vi "基于Lab颜色空间的自适应分割算法.vi"(11 "火焰占比系数":dbl(slide)=0.9 min=0.0 max=1.0 step=0.05 scale=0.0..1.0 scale format="%1.2f") -> ()   [LabVIEW 2018]
doc: "This example shows how to open, read, and display an AVI file in NI Vision. The VI reads the frames per second property and plays the images back at the rate specified by the AVI file."
uses:
  <vilib>/vision/NI_Vision_Development_Module.lvlib
  Dll/fire_Otsu.dll
panel:
  out "导入像素当量":bool
  in  "?":bool
  out "叠加实际字符串":string
  out "单帧实际字符串":string
  out "叠加像素字符串":string
  out "单帧像素字符串":string
  out "循环截止":bool
  in  "取消按钮":bool
  out "火焰帧数":string
  in  "单帧回看":bool
  out "叠加部分":string
  out "单帧部分":string
  in  "返回":bool
  out "火焰分割":T1(plugin-control)
  out "单幅画面":T1(plugin-control) caption="单帧画面"
  out "Progress Bar":i32(slide) max=241 scale=-1.1..241.0
  in  "程序停止":bool
  out "原图":T1(plugin-control)
  out "火焰叠加":T1(plugin-control)
  # "Lab颜色空间的最大类间方法火焰分割"
  # "火焰参数"
  # "参\n数\n设\n置"
  # "说明：\n火焰实际面积的单位为标定时的设定的单位，若未进行标注，则不显示实际尺寸。"
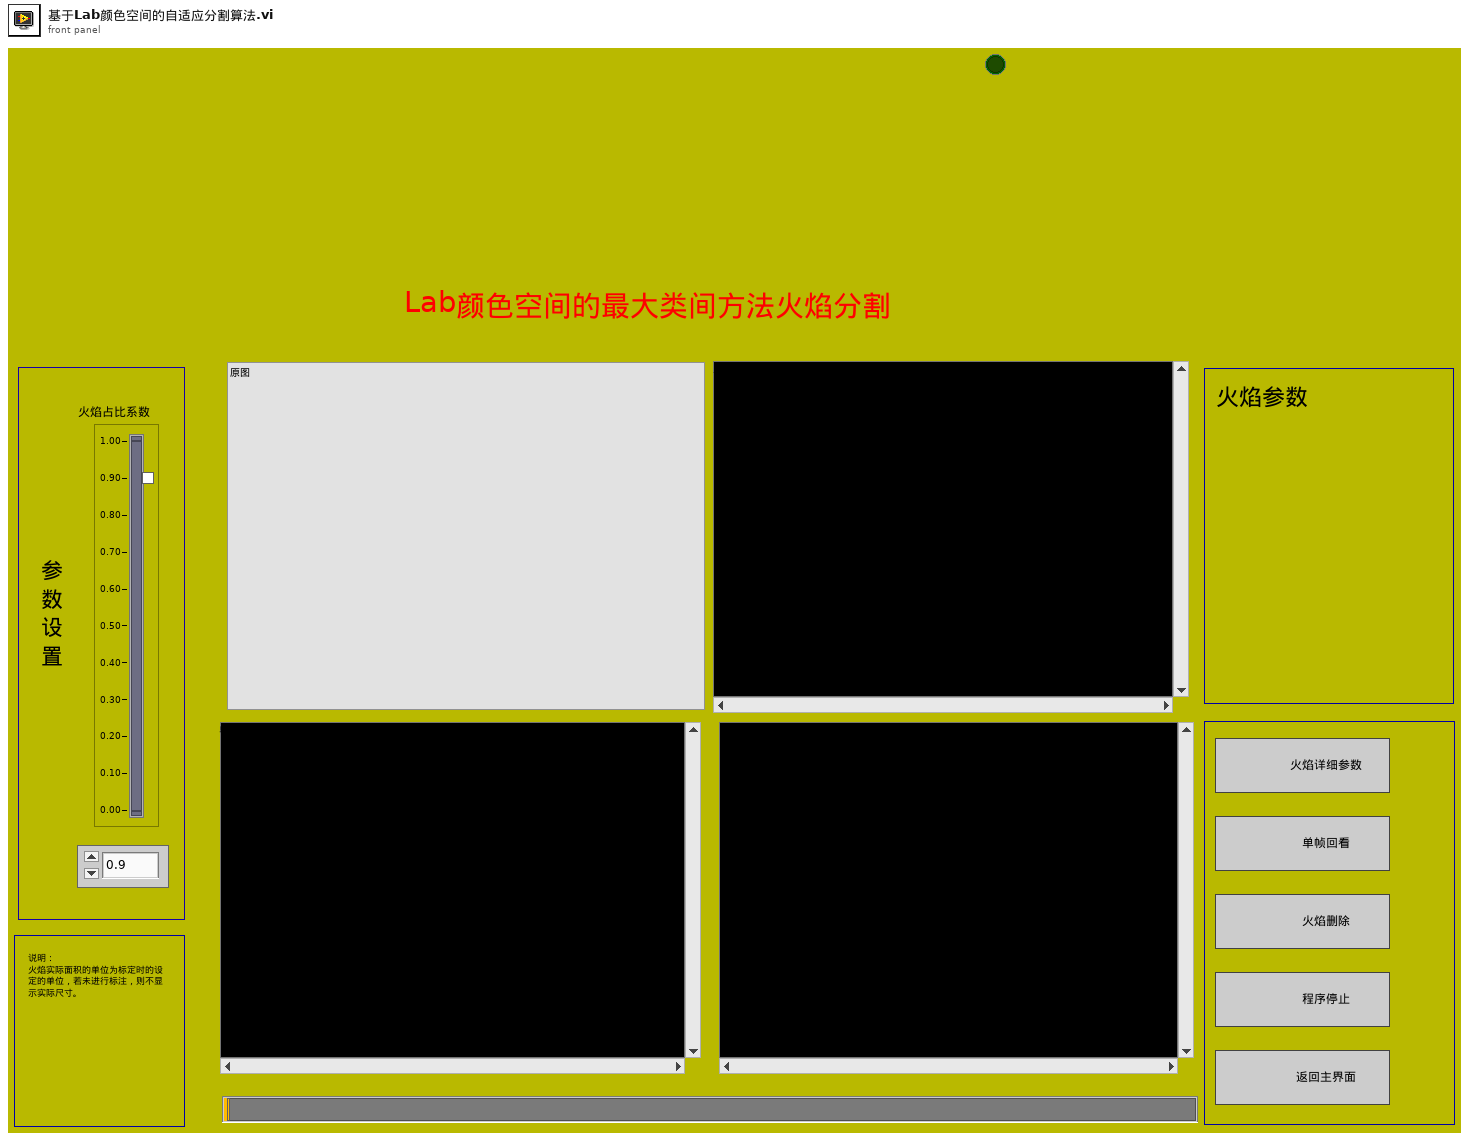
[diagram p1: front panel]
types:
  T1 = typedef "IMAQ Image.ctl" = refnum<image>
  T2 = enum8{"Enabled", "Disabled", "Disabled and Grayed Out"}
  T3 = cluster{"X Size":i32, "Y Size":i32, "% Tolerance":i32}
  T4 = enum32{"Invalid", "Standard", "Closed", "Hidden", "Minimized", "Maximized"}
  T5 = typedef "Image Type" = u32
  T6 = cluster{"Width":u32, "Height":u32, "Frames Per Second":u32, "Codec":string, "Has Data":bool}
  T7 = typedef "IMAQ AVI2 Refnum.ctl" = refnum<k20>
  T8 = typedef "ROI Descriptor" = cluster{"Global Rectangle":i32[], "Contours":cluster{"ID":enum32{"External", "Internal"}, "Type":u32, "Coordinates":i32[]}[]}
  T9 = cluster{"Area":dbl, "Number of Holes":dbl, "Bounding Rect":cluster{"Left":dbl, "Top":dbl, "Right":dbl, "Bottom":dbl}, "Center of Mass":cluster{"X":dbl, "Y":dbl}, "Orientation":dbl, "Dimensions":cluster{"Width":dbl, "Height":dbl}}[]
  T10 = cluster{"Particle Reports (Pixels)[0]":cluster{"Area":dbl, "Number of Holes":dbl, "Bounding Rect":cluster{"Left":dbl, "Top":dbl, "Right":dbl, "Bottom":dbl}, "Center of Mass":cluster{"X":dbl, "Y":dbl}, "Orientation":dbl, "Dimensions":cluster{"Width":dbl, "Height":dbl}}, "Particle Reports (Pixels)[1]":cluster{"Area":dbl, "Number of Holes":dbl, "Bounding Rect":cluster{"Left":dbl, "Top":dbl, "Right":dbl, "Bottom":dbl}, "Center of Mass":cluster{"X":dbl, "Y":dbl}, "Orientation":dbl, "Dimensions":cluster{"Width":dbl, "Height":dbl}}, "Particle Reports (Pixels)[2]":cluster{"Area":dbl, "Number of Holes":dbl, "Bounding Rect":cluster{"Left":dbl, "Top":dbl, "Right":dbl, "Bottom":dbl}, "Center of Mass":cluster{"X":dbl, "Y":dbl}, "Orientation":dbl, "Dimensions":cluster{"Width":dbl, "Height":dbl}}, "Particle Reports (Pixels)[3]":cluster{"Area":dbl, "Number of Holes":dbl, "Bounding Rect":cluster{"Left":dbl, "Top":dbl, "Right":dbl, "Bottom":dbl}, "Center of Mass":cluster{"X":dbl, "Y":dbl}, "Orientation":dbl, "Dimensions":cluster{"Width":dbl, "Height":dbl}}, "Particle Reports (Pixels)[4]":cluster{"Area":dbl, "Number of Holes":dbl, "Bounding Rect":cluster{"Left":dbl, "Top":dbl, "Right":dbl, "Bottom":dbl}, "Center of Mass":cluster{"X":dbl, "Y":dbl}, "Orientation":dbl, "Dimensions":cluster{"Width":dbl, "Height":dbl}}, "Particle Reports (Pixels)[5]":cluster{"Area":dbl, "Number of Holes":dbl, "Bounding Rect":cluster{"Left":dbl, "Top":dbl, "Right":dbl, "Bottom":dbl}, "Center of Mass":cluster{"X":dbl, "Y":dbl}, "Orientation":dbl, "Dimensions":cluster{"Width":dbl, "Height":dbl}}, "Particle Reports (Pixels)[6]":cluster{"Area":dbl, "Number of Holes":dbl, "Bounding Rect":cluster{"Left":dbl, "Top":dbl, "Right":dbl, "Bottom":dbl}, "Center of Mass":cluster{"X":dbl, "Y":dbl}, "Orientation":dbl, "Dimensions":cluster{"Width":dbl, "Height":dbl}}, "Particle Reports (Pixels)[7]":cluster{"Area":dbl, "Number of Holes":dbl, "Bounding Rect":cluster{"Left":dbl, "Top":dbl, "Right":dbl, "Bottom":dbl}, "Center of Mass":cluster{"X":dbl, "Y":dbl}, "Orientation":dbl, "Dimensions":cluster{"Width":dbl, "Height":dbl}}, "Particle Reports (Pixels)[8]":cluster{"Area":dbl, "Number of Holes":dbl, "Bounding Rect":cluster{"Left":dbl, "Top":dbl, "Right":dbl, "Bottom":dbl}, "Center of Mass":cluster{"X":dbl, "Y":dbl}, "Orientation":dbl, "Dimensions":cluster{"Width":dbl, "Height":dbl}}}
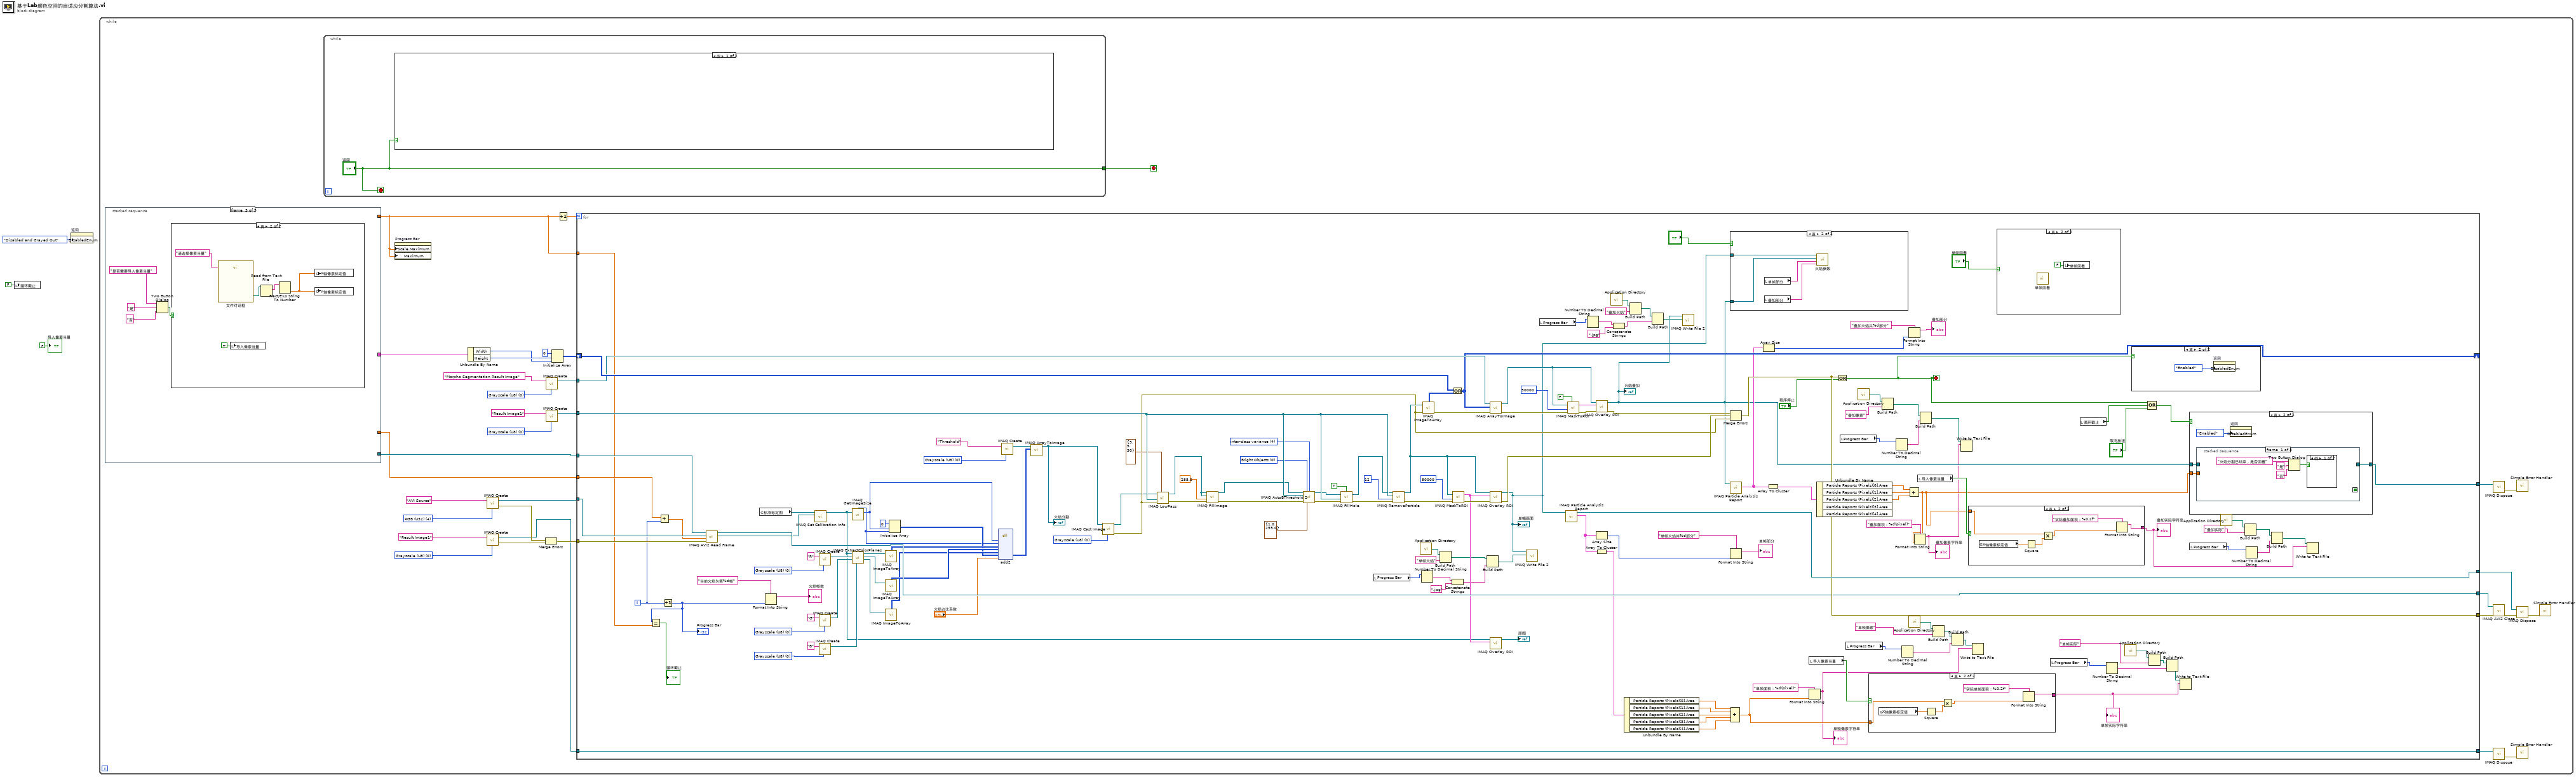
[diagram p0: block diagram]
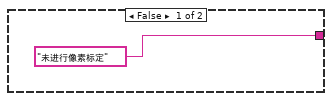
[diagram p3: hidden frame]
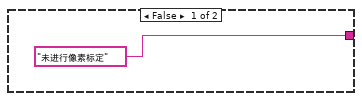
[diagram p4: hidden frame]
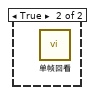
[diagram p7: hidden frame]
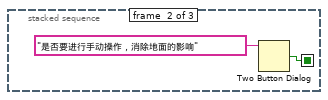
[diagram p8: hidden frame]
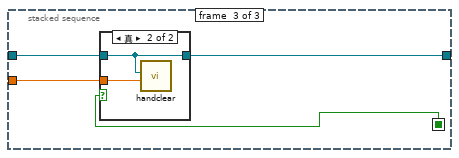
[diagram p9: hidden frame]
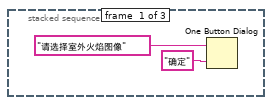
[diagram p12: hidden frame]
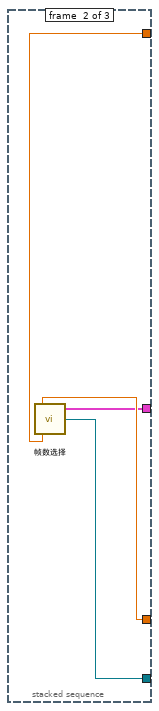
[diagram p13: hidden frame]
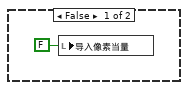
[diagram p14: hidden frame]
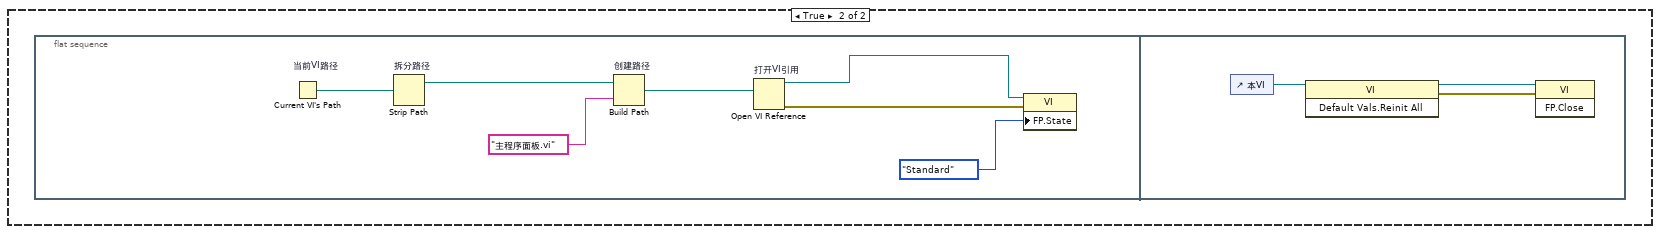
[diagram p15: hidden frame]
diagram:
  n1 = local write "循环截止"(FALSE ("循环截止")) -> ()
  n2 = property on="返回" class="Bool"("DisabledEnum"=T2."Disabled and Grayed Out" ("禁用")) -> ()  [unwired: 2 in, 2 out]
  n3 = while {
    stop <- w37 stop-if-true
    w24 = T5 0 items=["Grayscale (U8)", "Grayscale (I16)", "Grayscale (SGL)", "Complex (CSG)", "RGB (U32)", "HSL (U32)", "RGB (U64)", "Grayscale (U16)"] ("Image Type")
    w28 = T5 0 items=["Grayscale (U8)", "Grayscale (I16)", "Grayscale (SGL)", "Complex (CSG)", "RGB (U32)", "HSL (U32)", "RGB (U64)", "Grayscale (U16)"] ("Image Type")
    w30 = T5 0 items=["Grayscale (U8)", "Grayscale (I16)", "Grayscale (SGL)", "Complex (CSG)", "RGB (U32)", "HSL (U32)", "RGB (U64)", "Grayscale (U16)"] ("Image Type")
    w32 = T5 4 items=["Grayscale (U8)", "Grayscale (I16)", "Grayscale (SGL)", "Complex (CSG)", "RGB (U32)", "HSL (U32)", "RGB (U64)", "Grayscale (U16)"] ("Image Type")
    n4 = stacked-sequence {
      tunnel: [_ w239 _] -> w9
      tunnel: [_ w238 _] -> w5
      tunnel: [_ w237 _] -> w8
      tunnel: [_ w236 _] -> w7
      frame #0 {
        n5 = One Button Dialog(message="请选择室外火焰图像" ("消息"), button name ("OK")="确定" ("按钮名称（“确定”）")) -> ()  [unwired: 1 out]
      }
      frame #1 {
        n6 = call "帧数选择.vi"() -> ("请输入初始帧 2"=w237:dbl, "处理的总帧数 2"=w238:dbl, "Frame Data"=w236:T6, "AVI Refnum (duplicate)"=w239:T7)  [unwired: 1 out]
      }
      frame #2 {
        n7 = Two Button Dialog(message="是否需要导入像素当量" ("消息"), 1:"否" ("F按钮名称（“取消”）"), 2:"是" ("T按钮名称（“确定”）")) -> (T button?=w240:bool)
        n8 = case shown="真" w240 {
          frame False {
            n9 = local write "导入像素当量"(FALSE ("导入像素当量")) -> ()
          }
          frame True {
            n10 = call "文件对话框"("default name"="请选择像素当量") -> ("selected path"=w247:path)  [unwired: 11 in, 3 out]
            n11 = local write "导入像素当量"(TRUE ("导入像素当量")) -> ()
            n12 = Read from Text File(file (use dialog)=w247) -> (text=w248:string)  [unwired: 3 in, 3 out]
            n13 = Fract/Exp String To Number(string=w248) -> (number=w249:dbl)  [unwired: 3 in, 1 out]
            n14 = global write "全局变量.vi" "X轴像素标定值"(w249) -> ()
            n15 = global write "全局变量.vi" "Y轴像素标定值"(w249) -> ()
          }
        }
      }
    }
    n16 = while {
      tunnel: ["返回"] -> w37
      stop <- "返回" stop-if-true
      n17 = case shown="假" "返回" {
        frame False {
        }
        frame True {
          n18 = flat-sequence {
            frame #0 {
              n19 = Current VI's Path "当前VI路径"() -> (path=w255:path)
              n20 = Strip Path "拆分路径"(path=w255) -> (stripped path=w257:path)  [unwired: 1 out]
              n21 = Build Path "创建路径"(base path=w257, name or relative path="主程序面板.vi" ("名称或相对路径")) -> (appended path=w256:path)
              n22 = Open VI Reference "打开VI引用"(vi path=w256) -> (vi reference=w254:refnum<vi>, error out=w253:errorcluster)  [unwired: 5 in]
              n23 = property class="VI"(reference=w254, error in=w253, "FP.State"=T4."Standard" ("前面板窗口:状态")) -> ()  [unwired: 2 out]
            }
            frame #1 {
              n24 = control-ref of="本VI"() -> (w258:refnum<vi>)
              n25 = invoke class="VI" method="Default Vals.Reinit All"(reference=w258) -> (reference out=w259:refnum<vi>, error out=w260:errorcluster)  [unwired: 2 in, 1 out]
              n26 = invoke class="VI" method="FP.Close"(reference=w259, error in=w260) -> ()  [unwired: 1 in, 3 out]
            }
          }
        }
      }
    }
    n27 = property on="Progress Bar" class="Slide (严格)"("Scale.Maximum"=w5, "Maximum"=w5) -> ()  [unwired: 2 in, 2 out]
    n28 = Unbundle By Name(w7) -> ("Width"=w20:u32, "Height"=w21:u32)
    n29 = call "IMAQ Create"("Image Name"="AVI Source", "Image Type"=w32) -> ("New Image"=w33:T1, "error out"=w35:errorcluster)  [unwired: 2 in, 1 out]
    n30 = call "IMAQ Create"("Image Name"="Result Image1", "Image Type"=w24) -> ("New Image"=w23:T1, "error out"=w22:errorcluster)  [unwired: 2 in, 1 out]
    n31 = Merge Errors(w35, w22) -> (w34:errorcluster)
    n32 = call "IMAQ Create"("Image Name"="Morpho Segmentation Result Image", "Image Type"=w28) -> ("New Image"=w27:T1)  [unwired: 2 in, 2 out]
    n33 = call "IMAQ Create"("Image Name"="Result Image1", "Image Type"=w30) -> ("New Image"=w29:T1)  [unwired: 2 in, 2 out]
    n34 = Initialize Array(u8 0 ("元素"), w21, w20) -> (w18:u8[][])
    n35 = Increment(x=w5) -> (x+1=w4:dbl)
    n36 = for {
      N: w4 -> [_]
      tunnel: [w190] -> w16
      tunnel: [w192] -> w11
      tunnel: w34 -> [w188]
      tunnel: w33 -> [w189]
      tunnel: [w196] -> w13
      tunnel: w29 -> [w191]
      shift-right: [w193] -> _
      shift-left: w18 -> [w195]
      tunnel: w27 -> [w194]
      tunnel: w23 -> [w187]
      tunnel: [w187] -> w12
      tunnel: w9 -> [w108]
      tunnel: w8 -> [w107]
      tunnel: [w104] -> w6
      tunnel: w5 -> [w96]
      i -> [w99]
      stop <- w41 stop-if-true
      w136 = T5 0 items=["Grayscale (U8)", "Grayscale (I16)", "Grayscale (SGL)", "Complex (CSG)", "RGB (U32)", "HSL (U32)", "RGB (U64)", "Grayscale (U16)"] ("Image Type")
      w143 = T5 0 items=["Grayscale (U8)", "Grayscale (I16)", "Grayscale (SGL)", "Complex (CSG)", "RGB (U32)", "HSL (U32)", "RGB (U64)", "Grayscale (U16)"] ("Image Type")
      w144 = T5 0 items=["Grayscale (U8)", "Grayscale (I16)", "Grayscale (SGL)", "Complex (CSG)", "RGB (U32)", "HSL (U32)", "RGB (U64)", "Grayscale (U16)"] ("Image Type")
      w145 = T5 0 items=["Grayscale (U8)", "Grayscale (I16)", "Grayscale (SGL)", "Complex (CSG)", "RGB (U32)", "HSL (U32)", "RGB (U64)", "Grayscale (U16)"] ("Image Type")
      w179 = u32 0 items=["Bright Objects", "Dark Objects"] ("Look For (Bright Objects)")
      w182 = 4 items=["clustering", "entropy", "metric", "moments", "inter-class variance"] ("Method")
      w183 = T5 0 items=["Grayscale (U8)", "Grayscale (I16)", "Grayscale (SGL)", "Complex (CSG)", "RGB (U32)", "HSL (U32)", "RGB (U64)", "Grayscale (U16)"] ("Image Type")
      n37 = Add(x=w107, y=w99) -> (x+y=w130:dbl)
      n38 = Increment(x=w99) -> (x+1=w97:i32)
      "Progress Bar" <- w97
      n39 = Equal?(x=w97, y=w96) -> (x = y?=→"循环截止":bool)
      n40 = call "IMAQ AVI2 Read Frame"("error in (no error)"=w188, "Frame Number"=w130, "Image"=w189, "AVI Refnum"=w108) -> ("Image Out"=w101:T1, "AVI Refnum (duplicate)"=w190:T7)  [unwired: 6 out]
      n41 = global read "全局变量.vi" "标准标定图"() -> (w100:T1)
      n42 = Format Into String(format string="当前火焰为第%d帧" ("初始字符串"), w97) -> (resulting string=→"火焰帧数":string)  [unwired: 2 in, 1 out]
      n43 = call "IMAQ Set Calibration Info"("Image Dst"=w101, "Image Src"=w100) -> ("Calibrated Image"=w102:T1)  [unwired: 8 in, 1 out]
      n44 = call "IMAQ Create"("Image Name"="R", "Image Type"=w145) -> ("New Image"=w152:T1)  [unwired: 3 in, 1 out]
      n45 = call "IMAQ Create"("Image Name"="B", "Image Type"=w143) -> ("New Image"=w154:T1)  [unwired: 3 in, 1 out]
      n46 = call "IMAQ Create"("Image Name"="G", "Image Type"=w144) -> ("New Image"=w150:T1)  [unwired: 3 in, 1 out]
      n47 = call "IMAQ GetImageSize"("Image"=w102) -> ("Y Resolution"=w133:i32, "X Resolution"=w132:i32)  [unwired: 3 in, 1 out]
      n48 = call "IMAQ ExtractColorPlanes"("Blue or Luma or Val or Inten Plane"=w154, "Green or Sat Plane"=w150, "Red or Hue Plane"=w152, "Image Src"=w102) -> ("Blue or Luma or Val or Inten Plane out"=w146:T1, "Green or Sat Plane out"=w147:T1, "Red or Hue Plane out"=w148:T1)  [unwired: 4 in, 1 out]
      n49 = call "IMAQ ImageToArray"("Image"=w148) -> ("Image Pixels (U8)"=w140:u8[][])  [unwired: 3 in, 4 out]
      n50 = call "IMAQ ImageToArray"("Image"=w147) -> ("Image Pixels (U8)"=w142:u8[][])  [unwired: 3 in, 4 out]
      n51 = call "IMAQ ImageToArray"("Image"=w146) -> ("Image Pixels (U8)"=w141:u8[][])  [unwired: 3 in, 4 out]
      n52 = Initialize Array ("data")(u8 0, w133, w132) -> (w135:u8[][])
      n53 = dll-call lib="C:/Users/12435/Desktop/fire image processing/Dll/fire_Otsu.dll" fn="add2"("rows"=w133, "cols"=w132, "ImageR"=w140, "ImageG"=w142, "ImageB"=w141, "data"=w135, "a"="火焰占比系数") -> ("data"=w139:u8[][])  [unwired: 10 in, 2 out]
      n54 = call "IMAQ Create"("Image Name"="Threshold", "Image Type"=w136) -> ("New Image"=w138:T1)  [unwired: 3 in, 1 out]
      n55 = call "IMAQ ArrayToImage"("Image Pixels (U8)"=w139, "Image"=w138) -> ("Image Out"=w131:T1)  [unwired: 8 in, 1 out]
      "火焰分割" <- w131
      n56 = call "IMAQ Cast Image"("Image Type"=w183, "Image Src"=w131) -> ("error out"=w161:errorcluster, "Image Dst Out"=w156:T1)  [unwired: 8 in]
      n57 = call "IMAQ LowPass"("Image Src"=w156, "Size & Tolerance"=T3 {"X Size"=5, "Y Size"=5, "% Tolerance"=30}, "Image Dst"=w191, "error in (no error)"=w161) -> ("Image Dst Out"=w166:T1, "error out"=w170:errorcluster)  [unwired: 3 in]
      n58 = call "IMAQ FillImage"("error in (no error)"=w170, "Pixel Value (U8, U16, I16, Float)"=sgl 255.0, "Image Mask"=w166, "Image"=w166) -> ("error out"=w169:errorcluster, "Image Out"=w165:T1)  [unwired: 6 in]
      n59 = call "IMAQ AutoBThreshold 2"("Image Src"=w165, "Look For (Bright Objects)"=w179, "Method (clustering)"=w182, "Image Dst"=w191, "error in (no error)"=w169, "Threshold Limits"=cluster{"Lower value":sgl, "Upper value":sgl} {"Lower value"=1.0, "Upper value"=255.0}) -> ("Image Dst Out"=w168:T1, "error out"=w181:errorcluster)  [unwired: 2 in, 6 out]
      n60 = call "IMAQ FillHole"("error in (no error)"=w181, "Image Dst"=w191, "Image Src"=w168, "Connectivity 4/8 (8)"=TRUE) -> ("error out"=w177:errorcluster, "Image Dst Out"=w167:T1)  [unwired: 2 in]
      n61 = local read "Progress Bar"() -> (w85:i32)
      n62 = call "IMAQ RemoveParticle"("error in (no error)"=w177, "Number of Erosion"=12, "Image Dst"=w191, "Image Src"=w167) -> ("error out"=w175:errorcluster, "Image Dst Out"=w164:T1)  [unwired: 6 in]
      n63 = call <vilib>:"Application Directory.vi"() -> ("Application Directory"=w94:path)
      n64 = Number To Decimal String(number=w85) -> (decimal integer string=w80:string)  [unwired: 1 in]
      n65 = call "IMAQ ImageToArray"("error in (no error)"=w161, "Image"=w164) -> ("error out"=w160:errorcluster, "Image Pixels (U8)"=w163:u8[][])  [unwired: 2 in, 3 out]
      n66 = Build Path(base path=w94, name or relative path="单帧火焰" ("名称或相对路径")) -> (appended path=w93:path)
      n67 = Or(x=w195, y=w163) -> (x .or. y?=w193:u8[][])
      n68 = Concatenate Strings(w80, ".jpg" ("字符串")) -> (w79:string)
      n69 = call "IMAQ MaskToROI"("Image"=w164, "Max number of vectors in ROI"=50000, "error in (no error)"=w175) -> ("ROI Descriptor"=w110:T8, "error out"=w174:errorcluster)  [unwired: 4 in, 1 out]
      n70 = Build Path(base path=w93, name or relative path=w79) -> (appended path=w92:path)
      n71 = call "IMAQ ArrayToImage"("error in (no error)"=w160, "Image Pixels (U8)"=w193, "Image"=w194) -> ("error out"=w159:errorcluster, "Image Out"=w157:T1)  [unwired: 7 in]
      n72 = call "IMAQ Overlay ROI"("error in (no error)"=w174, "ROI Descriptor"=w110, "Image"=w164) -> ("error out"=w162:errorcluster, "Image Out"=w95:T1)  [unwired: 7 in]
      "单幅画面" <- w95
      n73 = call "IMAQ Overlay ROI"("ROI Descriptor"=w110, "Image"=w102) -> ("Image Out"=→"原图":T1)  [unwired: 8 in, 1 out]
      n74 = call-poly "IMAQ Write File 2"("File Path"=w92, "Image"=w95) -> ()  [unwired: 8 in, 2 out]
      n75 = local read "Progress Bar"() -> (w84:i32)
      n76 = call "IMAQ Particle Analysis Report"("Image"=w95) -> ("Particle Reports (Pixels)"=w115:T9, "Image Out (duplicate)"=w196:T1)  [unwired: 5 in, 4 out]
      n77 = call "IMAQ MaskToROI"("External edges only (T)"=FALSE, "Image"=w157, "Max number of vectors in ROI"=50000, "error in (no error)"=w159) -> ("ROI Descriptor"=w186:T8, "error out"=w185:errorcluster)  [unwired: 3 in, 1 out]
      n78 = Number To Decimal String(number=w84) -> (decimal integer string=w83:string)  [unwired: 1 in]
      n79 = Array To Cluster(array=w115) -> (cluster=w129:T10)
      n80 = call "IMAQ Overlay ROI"("error in (no error)"=w185, "ROI Descriptor"=w186, "Image"=w157) -> ("error out"=w158:errorcluster, "Image Out"=w86:T1)  [unwired: 7 in]
      "火焰叠加" <- w86
      n81 = Array Size(array=w115) -> (size(s)=w118:i32)
      n82 = call <vilib>:"Application Directory.vi"() -> ("Application Directory"=w90:path)
      n83 = Concatenate Strings(w83, ".jpg" ("字符串")) -> (w82:string)
      n84 = Unbundle By Name(w129) -> ("Particle Reports (Pixels)[0].Area"=w128:dbl, "Particle Reports (Pixels)[1].Area"=w127:dbl, "Particle Reports (Pixels)[2].Area"=w126:dbl, "Particle Reports (Pixels)[3].Area"=w123:dbl, "Particle Reports (Pixels)[4].Area"=w122:dbl)
      n85 = Build Path(base path=w90, name or relative path="叠加火焰" ("名称或相对路径")) -> (appended path=w88:path)
      n86 = Build Path(base path=w88, name or relative path=w82) -> (appended path=w87:path)
      n87 = call-poly "IMAQ Write File 2"("File Path"=w87, "Image"=w86) -> ()  [unwired: 8 in, 2 out]
      n88 = case shown="真" "?" {
        tunnel: w86 -> [_ w233]
        tunnel: w95 -> [_ w230]
        frame False {
        }
        frame True {
          n89 = local read "单帧部分"() -> (w232:string)
          n90 = local read "叠加部分"() -> (w231:string)
          n91 = call "火焰参数.vi"(8:w231, 9:w232, "Image 2"=w233, "Image"=w230) -> ()  [unwired: 8 in]
        }
      }
      n92 = Merge Errors(w158, w162, w161) -> (w192:errorcluster)
      n93 = call "IMAQ Particle Analysis Report"("Image"=w86) -> ("Particle Reports (Pixels)"=w111:T9)  [unwired: 5 in, 5 out]
      n94 = Format Into String(format string="单帧火焰共%d部分" ("初始字符串"), w118) -> (resulting string=→"单帧部分":string)  [unwired: 2 in, 1 out]
      n95 = Compound Arithmetic op=ADD(w128, w127, w126, w123, w122) -> (w74:dbl)
      n96 = Array Size(array=w111) -> (size(s)=w113:i32)
      n97 = Array To Cluster(array=w111) -> (cluster=w125:T10)
      n98 = Format Into String(format string="单帧面积：%d(pixel)" ("格式字符串"), w74) -> (resulting string=w64:string)  [unwired: 2 in, 1 out]
      "单帧像素字符串" <- w64
      n99 = local read "导入像素当量"() -> (w75:bool)
      n100 = Unbundle By Name(w125) -> ("Particle Reports (Pixels)[0].Area"=w121:dbl, "Particle Reports (Pixels)[1].Area"=w120:dbl, "Particle Reports (Pixels)[2].Area"=w119:dbl)  [unwired: 2 out]
      n101 = Or(x=w192, y="程序停止") -> (x .or. y?=w41:bool)
      n102 = local read "Progress Bar"() -> (w62:i32)
      n103 = local read "Progress Bar"() -> (w66:i32)
      n104 = call <vilib>:"Application Directory.vi"() -> ("Application Directory"=w63:path)
      n105 = case shown="真" w75 {
        tunnel: ["未进行像素标定" w210] -> w67
        tunnel: w74 -> [_ w208]
        frame False {
        }
        frame True {
          n106 = global read "全局变量.vi" "X轴像素标定值"() -> (w207:dbl)
          n107 = Square(x=w207) -> (x^2=w209:dbl)
          n108 = Multiply(x=w208, y=w209) -> (x*y=w206:dbl)
          n109 = Format Into String(format string="实际单帧面积：%0.2f" ("格式字符串"), w206) -> (resulting string=w210:string)  [unwired: 2 in, 1 out]
        }
      }
      "单帧实际字符串" <- w67
      n110 = Build Path(base path=w63, name or relative path="叠加像素" ("字符串")) -> (appended path=w56:path)
      n111 = Number To Decimal String(number=w62) -> (decimal integer string=w54:string)  [unwired: 1 in]
      n112 = Number To Decimal String(number=w66) -> (decimal integer string=w42:string)  [unwired: 1 in]
      n113 = Format Into String(format string="叠加火焰共%d部分" ("初始字符串"), w113) -> (resulting string=→"叠加部分":string)  [unwired: 2 in, 1 out]
      n114 = call <vilib>:"Application Directory.vi"() -> ("Application Directory"=w65:path)
      n115 = Compound Arithmetic op=ADD(w121, w120, w119) -> (w72:dbl)
      n116 = Format Into String(format string="叠加面积：%d(pixel)" ("格式字符串"), w72) -> (resulting string=w61:string)  [unwired: 2 in, 1 out]
      "叠加像素字符串" <- w61
      n117 = local read "导入像素当量"() -> (w73:bool)
      n118 = Build Path(base path=w56, name or relative path=w54) -> (appended path=w55:path)
      n119 = Build Path(base path=w65, name or relative path="单帧像素" ("字符串")) -> (appended path=w43:path)
      n120 = Build Path(base path=w43, name or relative path=w42) -> (appended path=w44:path)
      n121 = Write to Text File(file (use dialog)=w55, text=w61) -> ()  [unwired: 2 in, 3 out]
      n122 = case shown="真" w73 {
        tunnel: ["未进行像素标定" w203] -> w58
        tunnel: w72 -> [_ w200]
        frame False {
        }
        frame True {
          n123 = global read "全局变量.vi" "X轴像素标定值"() -> (w201:dbl)
          n124 = Square(x=w201) -> (x^2=w202:dbl)
          n125 = Multiply(x=w200, y=w202) -> (x*y=w199:dbl)
          n126 = Format Into String(format string="实际叠加面积：%0.2f" ("格式字符串"), w199) -> (resulting string=w203:string)  [unwired: 2 in, 1 out]
        }
      }
      "叠加实际字符串" <- w58
      n127 = Write to Text File(file (use dialog)=w44, text=w64) -> ()  [unwired: 2 in, 3 out]
      n128 = case shown="真" "单帧回看" {
        frame False {
        }
        frame True {
          n129 = call "单帧回看.vi"() -> ()  [unwired: 28 in]
          n130 = local write "单帧回看"(FALSE ("单帧回看")) -> ()
        }
      }
      n131 = local read "Progress Bar"() -> (w68:i32)
      n132 = local read "循环截止"() -> (w40:bool)
      n133 = Number To Decimal String(number=w68) -> (decimal integer string=w48:string)  [unwired: 1 in]
      n134 = call <vilib>:"Application Directory.vi"() -> ("Application Directory"=w69:path)
      n135 = case shown="真" w41 {
        frame False {
        }
        frame True {
          n136 = property on="返回" class="Bool"("DisabledEnum"=T2."Enabled" ("禁用")) -> ()  [unwired: 2 in, 2 out]
        }
      }
      n137 = Compound Arithmetic op=OR ("复合运算")(w41, w40, "取消按钮") -> (w38:bool)
      n138 = Build Path(base path=w69, name or relative path="单帧实际" ("字符串")) -> (appended path=w49:path)
      n139 = Build Path(base path=w49, name or relative path=w48) -> (appended path=w46:path)
      n140 = Write to Text File(file (use dialog)=w46, text=w67) -> ()  [unwired: 2 in, 3 out]
      n141 = case shown="真" w38 {
        tunnel: w72 -> [_ w216]
        tunnel: w86 -> [_ w215]
        tunnel: [_ w214] -> w104
        frame False {
        }
        frame True {
          n142 = stacked-sequence {
            seq-local: [_ w221 _] -> [_ _ w226]
            tunnel: w215 -> [_ _ w225]
            tunnel: [_ _ w224] -> w214
            tunnel: w216 -> [_ _ w223]
            frame #0 {
              n143 = Two Button Dialog(message="火焰分割已结束，是否回看" ("消息"), 1:"否" ("F按钮名称（“取消”）"), 2:"是" ("T按钮名称（“确定”）")) -> (T button?=w220:bool)
              n144 = case shown="假" w220 {
                frame False {
                }
                frame True {
                  n145 = call "单帧回看.vi"() -> ()  [unwired: 28 in]
                }
              }
            }
            frame #1 {
              n146 = Two Button Dialog(message="是否要进行手动操作，消除地面的影响" ("消息")) -> (T button?=w221:bool)  [unwired: 2 in]
            }
            frame #2 {
              n147 = case shown="真" w226 {
                tunnel: w225 -> [w227 w229]
                tunnel: [w227 w229] -> w224
                tunnel: w223 -> [_ w228]
                frame False {
                }
                frame True {
                  n148 = call "handclear.vi"("总像素"=w228, "Image 3"=w229) -> ()  [unwired: 10 in]
                }
              }
            }
          }
          n149 = property on="返回" class="Bool"("DisabledEnum"=T2."Enabled" ("禁用")) -> ()  [unwired: 2 in, 2 out]
        }
      }
      n150 = local read "Progress Bar"() -> (w60:i32)
      n151 = call <vilib>:"Application Directory.vi"() -> ("Application Directory"=w59:path)
      n152 = Build Path(base path=w59, name or relative path="叠加实际" ("字符串")) -> (appended path=w53:path)
      n153 = Number To Decimal String(number=w60) -> (decimal integer string=w51:string)  [unwired: 1 in]
      n154 = Build Path(base path=w53, name or relative path=w51) -> (appended path=w50:path)
      n155 = Write to Text File(file (use dialog)=w50, text=w58) -> ()  [unwired: 2 in, 3 out]
    }
    n156 = call "IMAQ Dispose"("Image"=w6) -> ("error out"=w10:errorcluster)  [unwired: 2 in, 3 out]
    n157 = call "IMAQ AVI2 Close"("error in (no error)"=w11, "AVI Refnum"=w16) -> ("error out"=w15:errorcluster)  [unwired: 9 out]
    n158 = call "IMAQ Dispose"("Image"=w12) -> ("error out"=w14:errorcluster)  [unwired: 2 in, 3 out]
    n159 = call <vilib>:"Simple Error Handler.vi"("error in (no error)"=w10) -> ()  [unwired: 1 in, 8 out]
    n160 = call "IMAQ Dispose"("Image"=w13, "error in (no error)"=w15) -> ("error out"=w17:errorcluster)  [unwired: 1 in, 3 out]
    n161 = call <vilib>:"Simple Error Handler.vi"("error in (no error)"=w14) -> ()  [unwired: 1 in, 8 out]
    n162 = call <vilib>:"Simple Error Handler.vi"("error in (no error)"=w17) -> ()  [unwired: 1 in, 8 out]
  }
  "导入像素当量" <- FALSE ("导入像素当量")
